vi "采配水自动流程.vi"(11 "参数":cluster{"是否启用仪器":bool}) -> ()   [LabVIEW 2016, in "PLC.lvlib"]
uses:
  PLC.lvlib
panel:
  out "枚举":enum16{"初始化", "采配水启动", "等待", "配水", "排水", "结束"}(ring)
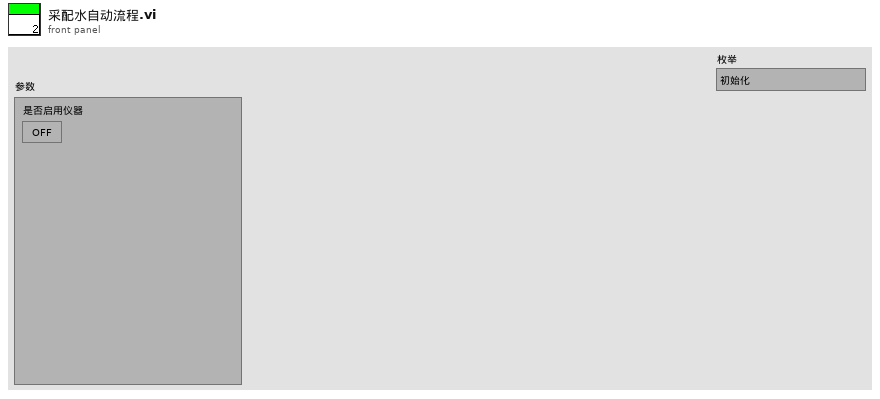
[diagram p1: front panel]
types:
  T1 = cluster{"命令":string, cluster{"starting address":u16, "holding register value":u16}}
  T2 = enum16{"待机", "启动氨氮", "氨氮测量中", "启动总磷", "总磷测量中", "结束"}
  T3 = enum16{"测量", "校零", "校标", "填充管路", "外部停止", "连续测量", "空白测量", "标样测量", "故障状态清除"}
  T4 = cluster{"站号":u16, "量程切换":enum32{"H", "L", "AUTO"}, "控制命令":enum16{"启动测量", "标样核查", "零点核查", "跨度核查", "空白测试", "平行样测试", "加标回收", "空白校准", "标样校准", "初始化（清洗）", "停止测试", "仪器重启", "校时", "模式设置", "测量间隔设置", "盲样测试"}, "模式设置":enum16{"待机", "连续模式", "周期模式", "定点模式", "受控模式", "手动模式"}, "测量间隔":u16}
  T5 = cluster{"时间标识":timestamp, "设备":string, "日志信息":string}
  T6 = cluster{"R0":i16, "R1":i16, "R2":i16, "R3":i16, "R4":i16, "R5":i16, "R6":i16, "R7":i16, "R8":i16, "R9":i16, "R10":i16, "R11":i16, "R12":i16, "R13":i16, "R14":i16, "R15":i16, "R16":i16, "R17":i16, "R18":i16, "R19":i16}
  T7 = cluster{"系统时间":timestamp, "工作状态":enum16{"空闲", "水样测试", "标样核查", "零点核查", "跨度核查", "空白测试", "平行样测试", "加标回收", "空白校准", "标样校准", "初始化（清洗）"}, "测量模式":enum16{"待机", "连续模式", "周期模式", "定点模式", "受控模式", "手动模式"}, "告警代码":enum16{"无告警", "缺试剂告警", "缺水样告警", "缺蒸馏水告警", "缺标液告警", "仪表漏液告警", "标定异常告警", "超量程告警", "加热异常", "低试剂预警", "超上限告警", "超下限告警", "仪表内部其他异常", "滴定异常告警", "电极异常告警", "量程切换告警", "参数设置告警", "PH电极电位异常", "电导率电极异常", "浊度光度异常", "溶解氧电极异常", "溶解氧光强异常", "温度异常告警", "PH异常告警", "溶解氧异常告警", "电导率异常告警", "浊度异常告警", "叶绿素异常告警", "藻密度异常告警", "蓝绿藻异常告警", "ORP异常告警", "氨氮异常告警", "清洁刷异常告警", "SD卡异常告警", "蓝牙异常告警", "Wifi异常告警", "流程异常告警"}, "故障代码":enum16{"无故障", "电机故障", "温度故障", "通讯故障", "滴定故障"}, "日志代码":u16, "软件版本":u16, "F0":sgl, "F1":sgl, "F2":sgl, "F3":sgl, "T":sgl, "H":sgl, "id":u16, "flowid":u16, "量程":u16}
  T8 = enum16{"空闲", "水样测试", "标样核查", "零点核查", "跨度核查", "空白测试", "平行样测试", "加标回收", "空白校准", "标样校准", "初始化（清洗）"}
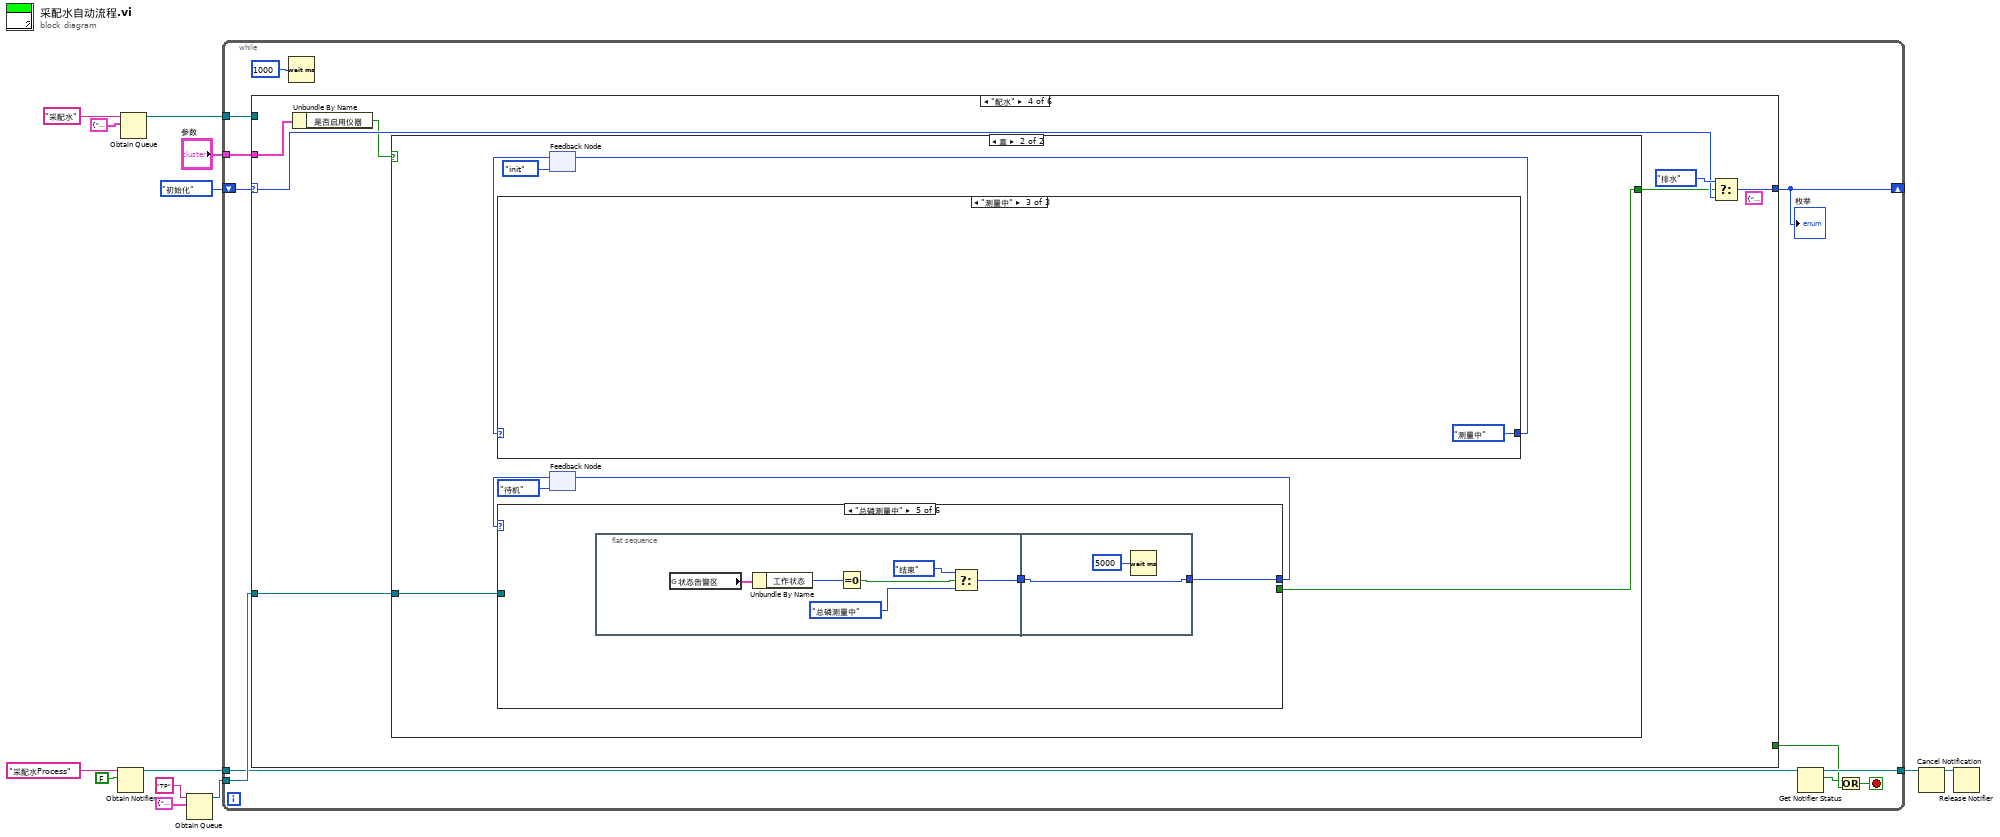
[diagram p0: block diagram]
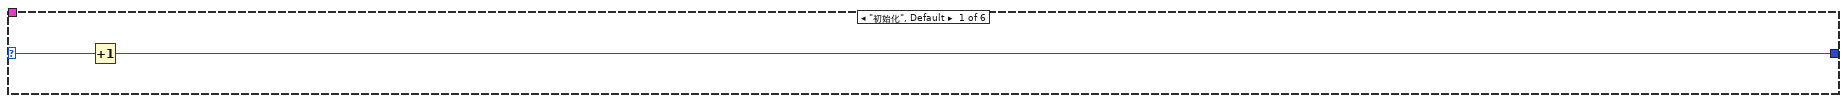
[diagram p2: hidden frame]
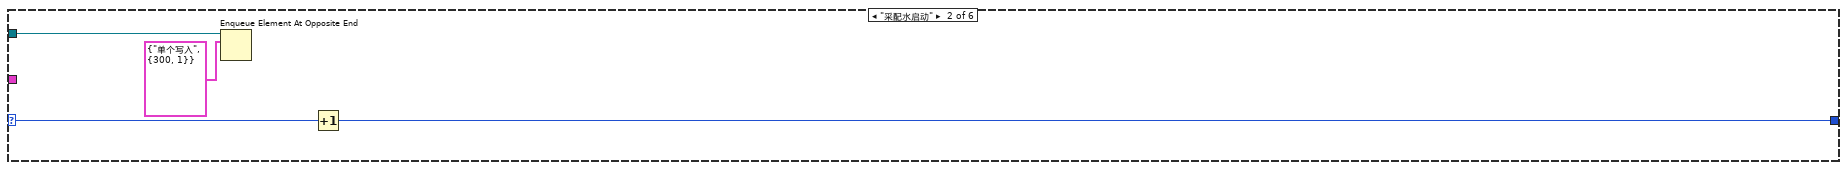
[diagram p3: hidden frame]
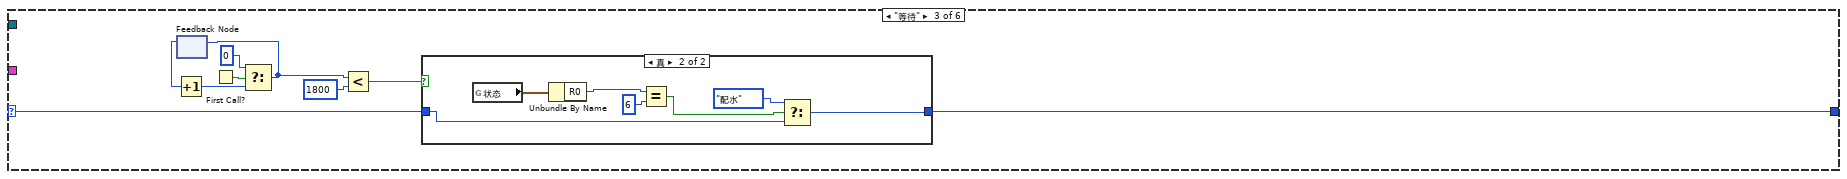
[diagram p4: hidden frame]
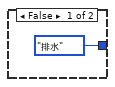
[diagram p5: hidden frame]
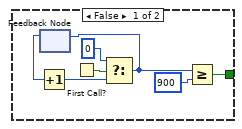
[diagram p6: hidden frame]
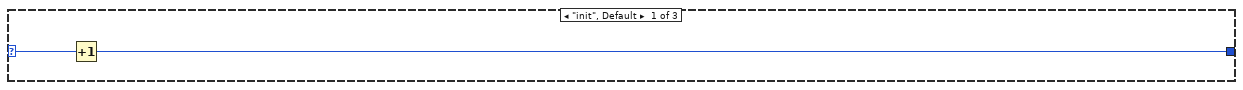
[diagram p7: hidden frame]
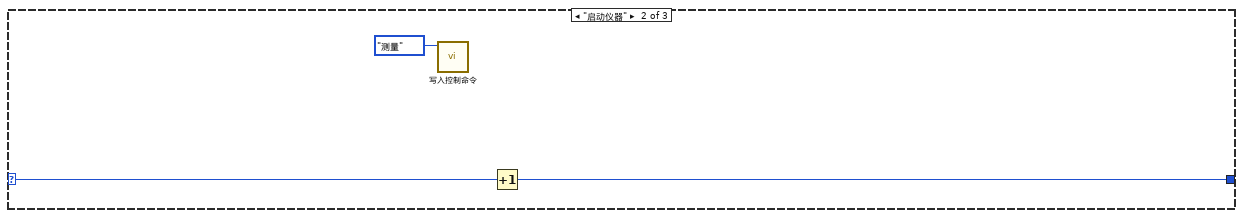
[diagram p8: hidden frame]
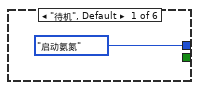
[diagram p9: hidden frame]
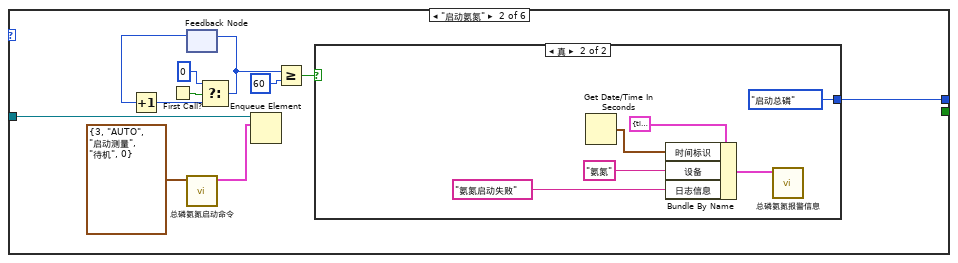
[diagram p10: hidden frame]
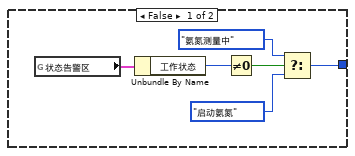
[diagram p11: hidden frame]
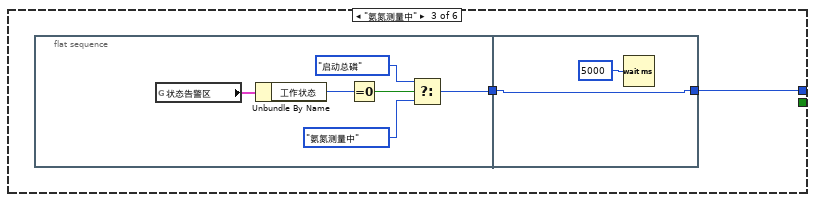
[diagram p12: hidden frame]
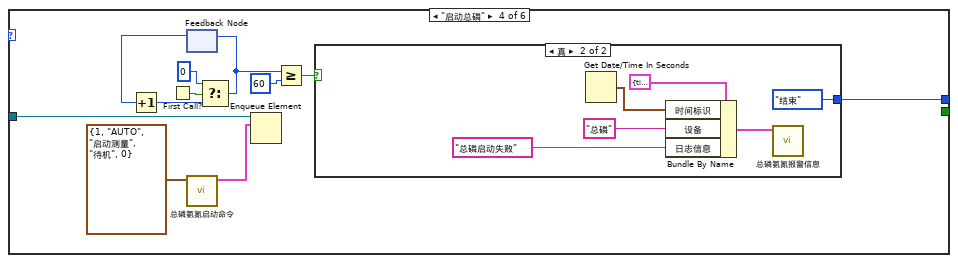
[diagram p13: hidden frame]
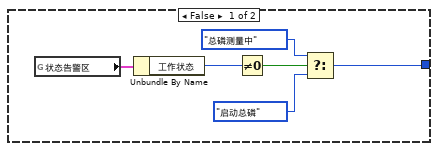
[diagram p14: hidden frame]
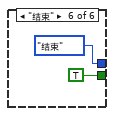
[diagram p15: hidden frame]
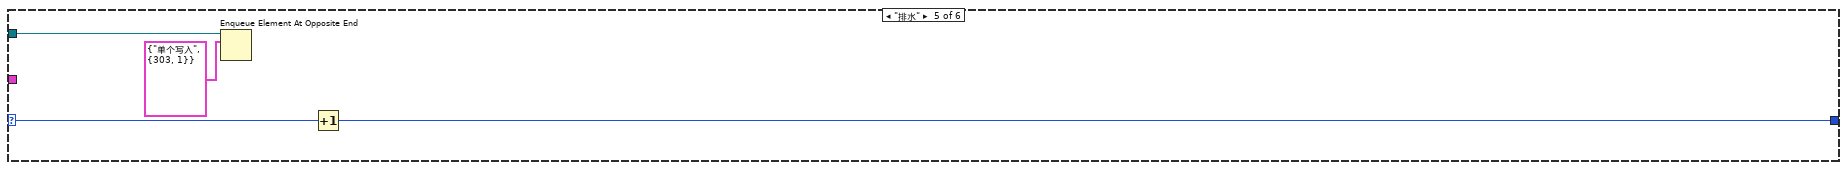
[diagram p16: hidden frame]
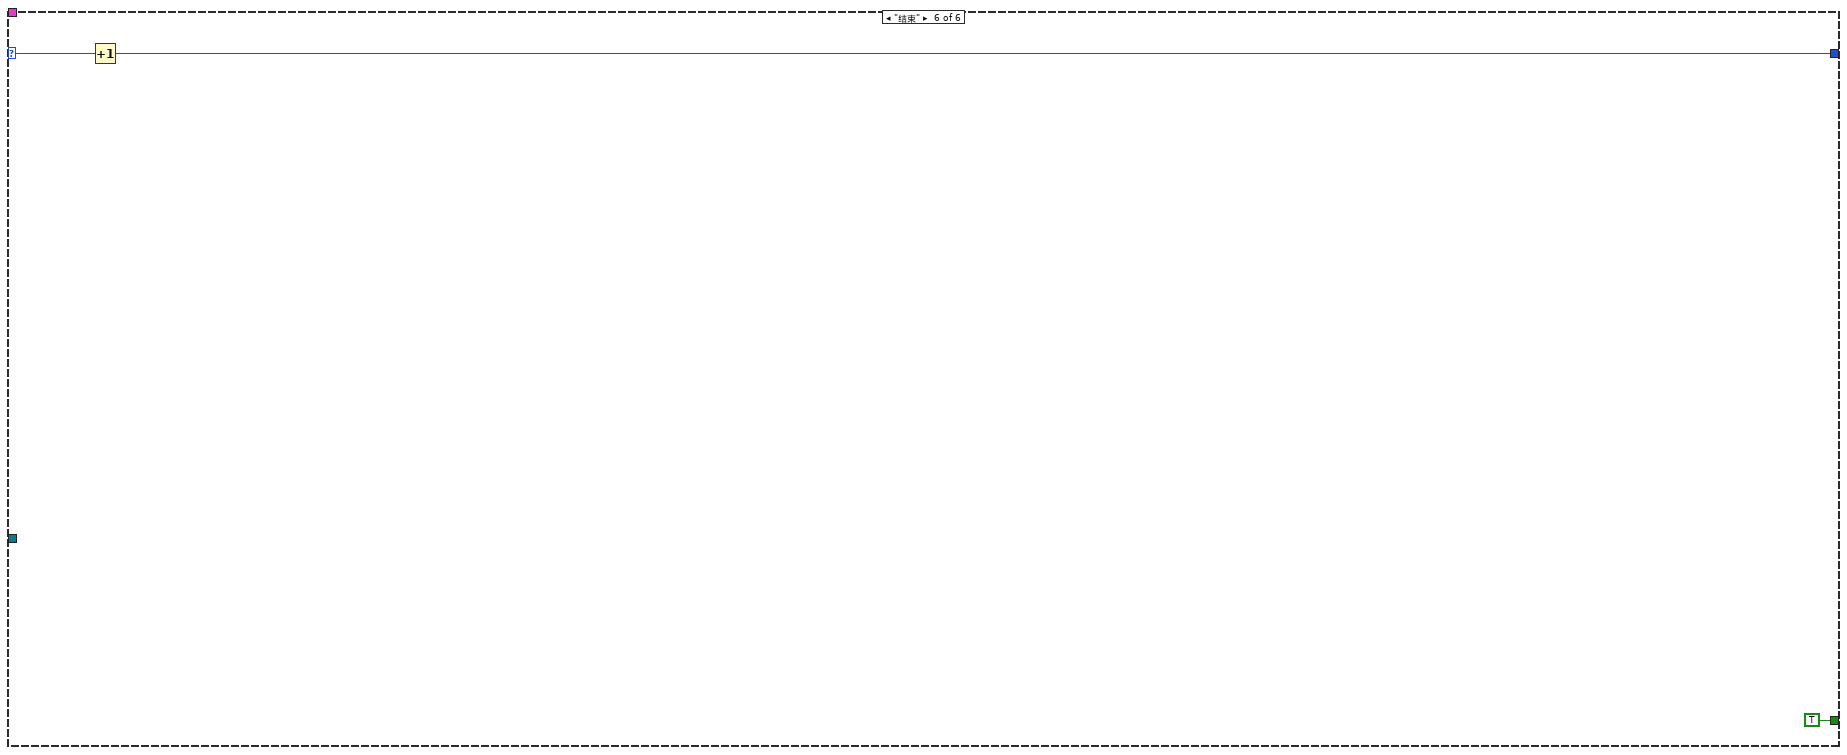
[diagram p17: hidden frame]
diagram:
  n1 = Obtain Notifier(name (unnamed)="采配水Process" ("名称（未命名）"), notification data type=FALSE) -> (notifier out=w3:refnum<notifier>)  [unwired: 2 in, 2 out]
  n2 = Obtain Queue(name (unnamed)="采配水" ("名称（未命名）"), element data type=cluster{"命令":string, "数据":variant} {"命令"="", "数据"=variant}) -> (queue out=w11:refnum<queue>)  [unwired: 3 in, 2 out]
  n3 = Obtain Queue(name (unnamed)="TP" ("名称（未命名）"), element data type=cluster{"命令":string, "data":variant} {"命令"="", "data"=variant}) -> (queue out=w7:refnum<queue>)  [unwired: 3 in, 2 out]
  n4 = while {
    tunnel: w11 -> [w24]
    shift-right: [w22] -> _
    shift-left: enum16{"初始化", "采配水启动", "等待", "配水", "排水", "结束"}."初始化" ("枚举") -> [w23]
    tunnel: w7 -> [w20]
    tunnel: "参数" -> [w19]
    tunnel: w3 -> [w18]
    tunnel: [w17] -> w2
    stop <- w16 stop-if-true
    n5 = case shown="\"配水\"" w23 {
      selector: w23 -> [w26 w28 w37 w53 w146 w151]
      tunnel: w24 -> [_ w29 _ _ w147 _]
      tunnel: [w25 w27 w36 w52 w145 w150] -> w22
      tunnel: [_ _ _ _ _ TRUE] -> w15
      tunnel: w20 -> [_ _ _ w51 _ _]
      tunnel: w19 -> [_ _ _ w50 _ _]
      frame "初始化", Default {
        n6 = Increment(x=w26) -> (x+1=w25:enum16{"初始化", "采配水启动", "等待", "配水", "排水", "结束"})
      }
      frame "采配水启动" {
        n7 = Enqueue Element At Opposite End(queue=w29, element=T1 {"命令"="单个写入", {"starting address"=300, "holding register value"=1}} ("元素")) -> ()  [unwired: 2 in, 3 out]
        n8 = Increment(x=w28) -> (x+1=w27:enum16{"初始化", "采配水启动", "等待", "配水", "排水", "结束"})
      }
      frame "等待" {
        n9 = feedback #1() -> (w33:i32)  [unwired: 1 in]
        n10 = Increment(x=w33) -> (x+1=w32:i32)
        n11 = First Call?() -> (First Call?: T/F=w34:bool)
        n12 = Select(t=0, s=w34, f=w32) -> (s? t:f=w31:i32)
        n13 = feedback-in #1(w31) -> ()
        n14 = Less?(x=w31, y=1800) -> (x < y?=w38:bool)
        n15 = case shown="真" w38 {
          tunnel: w37 -> [_ w42]
          tunnel: [enum16{"初始化", "采配水启动", "等待", "配水", "排水", "结束"}."排水" ("枚举") w41] -> w36
          frame False {
          }
          frame True {
            n16 = global read "采配水全局变量.vi" "状态"() -> (w47:T6)
            n17 = Unbundle By Name(w47) -> ("R0"=w46:i16)
            n18 = Equal?(x=w46, y=i16 6) -> (x = y?=w44:bool)
            n19 = Select(t=enum16{"初始化", "采配水启动", "等待", "配水", "排水", "结束"}."配水" ("枚举"), s=w44, f=w42) -> (s? t:f=w41:enum16{"初始化", "采配水启动", "等待", "配水", "排水", "结束"})
          }
        }
      }
      frame "配水" {
        (unwired) cluster{"命令":string, "data":variant} {"命令"="启动", "data"=variant(cluster{"站号":u16, "控制命令输出":u16[]} {"站号"=1, "控制命令输出"=[256, 0]})} ("元素")
        n20 = Unbundle By Name(w50) -> ("是否启用仪器"=w49:bool)
        n21 = case shown="真" w49 {
          tunnel: w51 -> [_ w66]
          tunnel: [w55 w65] -> w48
          frame False {
            n22 = feedback #2() -> (w59:i32)  [unwired: 1 in]
            n23 = Increment(x=w59) -> (x+1=w58:i32)
            n24 = First Call?() -> (First Call?: T/F=w60:bool)
            n25 = Select(t=0, s=w60, f=w58) -> (s? t:f=w56:i32)
            n26 = feedback-in #2(w56) -> ()
            n27 = Greater Or Equal?(x=w56, y=900) -> (x >= y?=w55:bool)
          }
          frame True {
            n28 = feedback #3(enum16{"init", "启动仪器", "测量中"}."init") -> (w63:enum16{"init", "启动仪器", "测量中"})
            n29 = case shown="\"测量中\"" w63 {
              selector: w63 -> [w71 w74 _]
              tunnel: [w70 w73 enum16{"init", "启动仪器", "测量中"}."测量中"] -> w64
              frame "init", Default {
                n30 = Increment(x=w71) -> (x+1=w70:enum16{"init", "启动仪器", "测量中"})
              }
              frame "启动仪器" {
                n31 = call "写入控制命令.vi"("命令"=T3."测量") -> ()  [unwired: 10 in, 1 out]
                n32 = Increment(x=w74) -> (x+1=w73:enum16{"init", "启动仪器", "测量中"})
              }
              frame "测量中" {
              }
            }
            n33 = feedback-in #3(w64) -> ()
            n34 = feedback #4(T2."待机") -> (w68:T2)
            n35 = case shown="\"总磷测量中\"" w68 {
              tunnel: [T2."启动氨氮" w86 w101 w119 w134 T2."结束"] -> w67
              tunnel: w66 -> [_ w87 _ w120 _ _]
              tunnel: [_ _ _ _ _ TRUE] -> w65
              frame "待机", Default {
              }
              frame "启动氨氮" {
                n36 = First Call?() -> (First Call?: T/F=w84:bool)
                n37 = feedback #5() -> (w83:i32)  [unwired: 1 in]
                n38 = Increment(x=w83) -> (x+1=w82:i32)
                n39 = call "总磷氨氮启动命令.vi"("参数"=T4 {"站号"=3, "量程切换"=enum."AUTO", "控制命令"=enum."启动测量", "模式设置"=enum."待机", "测量间隔"=0}) -> ("启动命令"=w78:cluster{"命令":string, "data":variant})  [unwired: 10 in]
                n40 = Select(t=0, s=w84, f=w82) -> (s? t:f=w81:i32)
                n41 = feedback-in #5(w81) -> ()
                n42 = Enqueue Element(queue=w87, element=w78) -> ()  [unwired: 2 in, 3 out]
                n43 = Greater Or Equal?(x=w81, y=60) -> (x >= y?=w79:bool)
                n44 = case shown="真" w79 {
                  tunnel: [w90 T2."启动总磷"] -> w86
                  frame False {
                    n45 = global read "VAR总磷氨氮全局变量.vi" "状态告警区"() -> (w93:T7)
                    n46 = Unbundle By Name(w93) -> ("工作状态"=w92:T8)
                    n47 = Not Equal To 0?(x=w92) -> (x != 0?=w91:bool)
                    n48 = Select(t=T2."氨氮测量中", s=w91, f=T2."启动氨氮") -> (s? t:f=w90:T2)
                  }
                  frame True {
                    n49 = Get Date/Time In Seconds() -> (seconds since 1Jan1904=w98:timestamp)
                    n50 = Bundle By Name(cluster=T5 {"时间标识"=timestamp(0 s since 1904-01-01), "设备"="", "日志信息"=""} ("data in"), "时间标识"=w98, "设备"="氨氮", "日志信息"="氨氮启动失败") -> (w94:T5)
                    n51 = call "总磷氨氮报警信息.vi"("data in"=w94) -> ()  [unwired: 11 in]
                  }
                }
              }
              frame "氨氮测量中" {
                n52 = flat-sequence {
                  tunnel: [w105] -> w100
                  tunnel: [w109] -> w101
                  tunnel: w100 -> [w109]
                  frame #0 {
                    n53 = global read "VAR总磷氨氮全局变量.vi" "状态告警区"() -> (w106:T7)
                    n54 = Unbundle By Name(w106) -> ("工作状态"=w107:T8)
                    n55 = Equal To 0?(x=w107) -> (x = 0?=w104:bool)
                    n56 = Select(t=T2."启动总磷", s=w104, f=T2."氨氮测量中") -> (s? t:f=w105:T2)
                  }
                  frame #1 {
                    n57 = Wait (ms)(milliseconds to wait=u32 5000 ("等待时间（毫秒）")) -> ()  [unwired: 1 out]
                  }
                }
              }
              frame "启动总磷" {
                n58 = First Call?() -> (First Call?: T/F=w117:bool)
                n59 = feedback #6() -> (w116:i32)  [unwired: 1 in]
                n60 = Increment(x=w116) -> (x+1=w115:i32)
                n61 = call "总磷氨氮启动命令.vi"("参数"=T4 {"站号"=1, "量程切换"=enum."AUTO", "控制命令"=enum."启动测量", "模式设置"=enum."待机", "测量间隔"=0}) -> ("启动命令"=w111:cluster{"命令":string, "data":variant})  [unwired: 10 in]
                n62 = Select(t=0, s=w117, f=w115) -> (s? t:f=w114:i32)
                n63 = feedback-in #6(w114) -> ()
                n64 = Enqueue Element(queue=w120, element=w111) -> ()  [unwired: 2 in, 3 out]
                n65 = Greater Or Equal?(x=w114, y=60) -> (x >= y?=w112:bool)
                n66 = case shown="真" w112 {
                  tunnel: [w123 T2."结束"] -> w119
                  frame False {
                    n67 = global read "VAR总磷氨氮全局变量.vi" "状态告警区"() -> (w124:T7)
                    n68 = Unbundle By Name(w124) -> ("工作状态"=w125:T8)
                    n69 = Not Equal To 0?(x=w125) -> (x != 0?=w126:bool)
                    n70 = Select(t=T2."总磷测量中", s=w126, f=T2."启动总磷") -> (s? t:f=w123:T2)
                  }
                  frame True {
                    n71 = Get Date/Time In Seconds() -> (seconds since 1Jan1904=w132:timestamp)
                    n72 = Bundle By Name(cluster=T5 {"时间标识"=timestamp(0 s since 1904-01-01), "设备"="", "日志信息"=""} ("data in"), "时间标识"=w132, "设备"="总磷", "日志信息"="总磷启动失败") -> (w128:T5)
                    n73 = call "总磷氨氮报警信息.vi"("data in"=w128) -> ()  [unwired: 11 in]
                  }
                }
              }
              frame "总磷测量中" {
                n74 = flat-sequence {
                  tunnel: [w138] -> w133
                  tunnel: [w142] -> w134
                  tunnel: w133 -> [w142]
                  frame #0 {
                    n75 = global read "VAR总磷氨氮全局变量.vi" "状态告警区"() -> (w139:T7)
                    n76 = Unbundle By Name(w139) -> ("工作状态"=w140:T8)
                    n77 = Equal To 0?(x=w140) -> (x = 0?=w137:bool)
                    n78 = Select(t=T2."结束", s=w137, f=T2."总磷测量中") -> (s? t:f=w138:T2)
                  }
                  frame #1 {
                    n79 = Wait (ms)(milliseconds to wait=u32 5000 ("等待时间（毫秒）")) -> ()  [unwired: 1 out]
                  }
                }
              }
              frame "结束" {
              }
            }
            n80 = feedback-in #4(w67) -> ()
          }
        }
        n81 = Select(t=enum16{"初始化", "采配水启动", "等待", "配水", "排水", "结束"}."排水" ("枚举"), s=w48, f=w53) -> (s? t:f=w52:enum16{"初始化", "采配水启动", "等待", "配水", "排水", "结束"})
      }
      frame "排水" {
        n82 = Enqueue Element At Opposite End(queue=w147, element=T1 {"命令"="单个写入", {"starting address"=303, "holding register value"=1}} ("元素")) -> ()  [unwired: 2 in, 3 out]
        n83 = Increment(x=w146) -> (x+1=w145:enum16{"初始化", "采配水启动", "等待", "配水", "排水", "结束"})
      }
      frame "结束" {
        n84 = Increment(x=w151) -> (x+1=w150:enum16{"初始化", "采配水启动", "等待", "配水", "排水", "结束"})
      }
    }
    "枚举" <- w22
    n85 = Wait (ms)(milliseconds to wait=u32 1000 ("等待时间（毫秒）")) -> ()  [unwired: 1 out]
    n86 = Get Notifier Status(notifier=w18) -> (notifier out=w17:refnum<notifier>, current notification=w14:bool)  [unwired: 1 in, 3 out]
    n87 = Or(x=w14, y=w15) -> (x .or. y?=w16:bool)
  }
  n88 = Cancel Notification(0:w2) -> (8:w1:refnum<notifier>)  [unwired: 1 in, 2 out]
  n89 = Release Notifier(notifier=w1) -> ()  [unwired: 2 in, 3 out]
